vi "Initialize with checks.vi"(5 "Password":string, 6 "Force online? (true)":bool=TRUE, 7 "Username":string, 8 "error in (no error)":errorcluster, 11 "System Session in":refnum<k21>) -> (0 "error out":errorcluster, 3 "System Session out":refnum<k21>)   [LabVIEW 2016, in "RT Management.lvlib" / "RT Management.lvclass"]
doc: "Initalize the System Configuration session with two checks: that the target is online and is an RT target. The former is an optional check and the latter is required."
uses:
  RT Management.lvclass
  <vilib>/nisyscfg/nisyscfg.lvlib
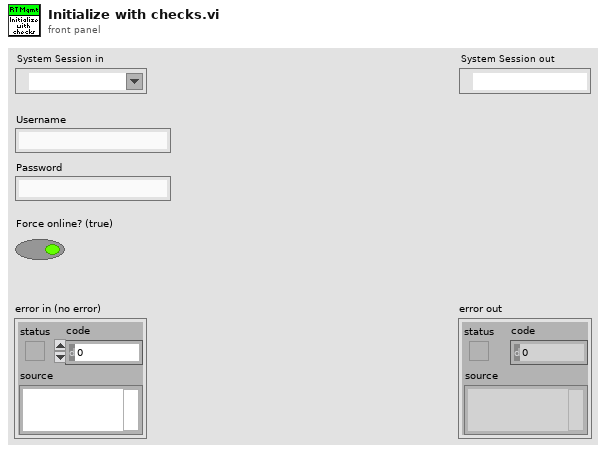
[diagram p1: front panel]
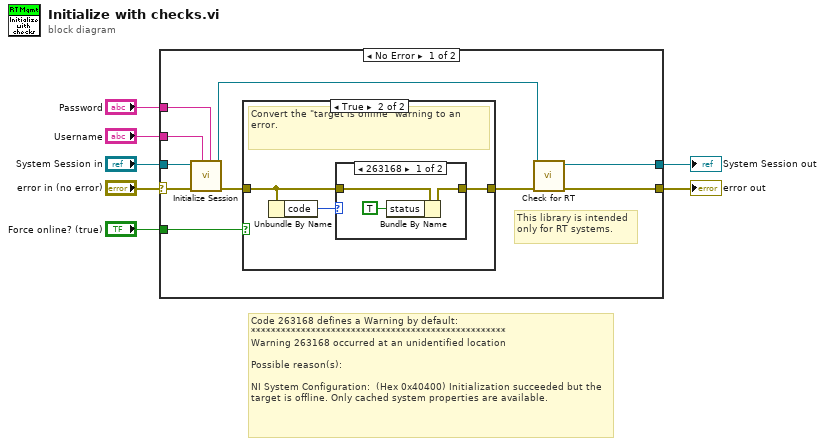
[diagram p0: block diagram]
diagram:
  # "Code 263168 defines a Warning by default:\n***************************************************\nWarning 263168 occurred at an unidentified location\n\nPossible reason(s):\n\nNI System Configuration:  (Hex 0x40400) Initialization succeeded but the target is offline. Only cached system properties are available."
  n1 = case shown="No Error" "error in (no error)" {
    selector: "error in (no error)" -> [w17 w27]
    tunnel: [w12 w27] -> w6
    tunnel: "System Session in" -> [w16 w26]
    tunnel: [w11 w26] -> w4
    tunnel: "Force online? (true)" -> [w14 _]
    tunnel: "Username" -> [w9 _]
    tunnel: "Password" -> [w8 _]
    frame No Error {
      # "This library is intended only for RT systems."
      n2 = call <vilib>:"Initialize Session.vi"("Password"=w8, "User Name"=w9, "error in (no error)"=w17, "Target (localhost)"=w16) -> ("error out"=w15:errorcluster, "Session out"=w10:refnum<k21>)  [unwired: 6 in]
      n3 = case shown="True" w14 {
        tunnel: w15 -> [w18 w20]
        tunnel: [w18 w19] -> w13
        frame False {
        }
        frame True {
          # "Convert the \"target is offline\" warning to an error."
          n4 = Unbundle By Name(w20) -> ("code"=w21:i32)
          n5 = case shown="263168" w21 {
            tunnel: w20 -> [w23 w25]
            tunnel: [w22 w25] -> w19
            frame 263168 {
              n6 = Bundle By Name(cluster=w23, "status"=TRUE) -> (w22:errorcluster)
            }
            frame Default {
            }
          }
        }
      }
      n7 = call "Check for RT.vi"("error in (no error)"=w13, "System Session in"=w10) -> ("error out"=w12:errorcluster, "System Session out"=w11:refnum<k21>)  [unwired: 8 in]
    }
    frame Error {
    }
  }
  "error out" <- w6
  "System Session out" <- w4
